vi "Floating Intake Teleop.vi"(11 "Cluster":T1) -> ()   [LabVIEW 2018]
uses:
  Support Code/Joystick Vals.ctl
  <vilib>/Rock Robotics/Network Tables/NT Read Boolean.vi
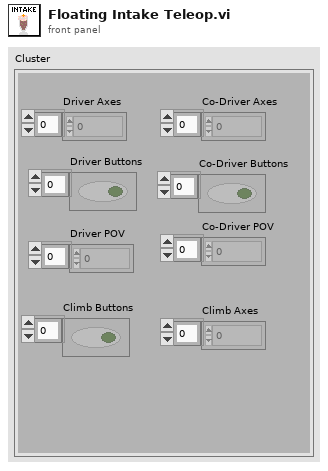
[diagram p1: front panel]
types:
  T1 = typedef "Joystick Vals.ctl" = cluster{"Driver Axes":dbl[], "Co-Driver Axes":dbl[], "Driver Buttons":bool[], "Co-Driver Buttons":bool[], "Driver POV":i16[], "Co-Driver POV":i16[], "Climb Buttons":bool[], "Climb Axes":dbl[]}
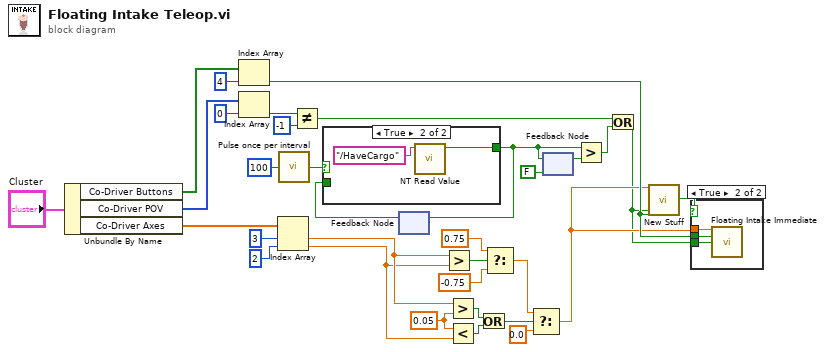
[diagram p0: block diagram]
diagram:
  w8 = 0.05 ("y")
  n1 = Unbundle By Name("Cluster") -> ("Co-Driver Buttons"=w30:bool[], "Co-Driver POV"=w26:i16[], "Co-Driver Axes"=w25:dbl[])
  n2 = Index Array(array=w30, index=4) -> (element=w15:bool)
  n3 = Index Array(array=w26, index=0) -> (element=w23:i16)
  n4 = Index Array(array=w25, index #1=3 ("index"), index #2=2 ("index")) -> (element #1=w14:dbl, element #2=w13:dbl)
  n5 = call "Pulse once per interval.vi"("Time (ms)"=u32 100 ("y")) -> ("Boolean"=w12:bool)
  n6 = Not Equal?(x=w23, y=i16 -1) -> (x != y?=w22:bool)
  n7 = feedback #1() -> (w17:bool)  [unwired: 1 in]
  n8 = case shown="True" w12 {
    tunnel: [w34 w36] -> w18
    tunnel: w17 -> [w34 _]
    frame False {
    }
    frame True {
      n9 = call-poly <vilib>:"NT Read Value.vi"("Name"="/HaveCargo") -> ("Boolean"=w36:bool)  [unwired: 9 in, 1 out]
    }
  }
  n10 = feedback-in #1(w18) -> ()
  n11 = Greater?(x=w14, y=w13) -> (0:w5:bool)
  n12 = Greater?(x=w14, y=w8) -> (0:w9:bool)
  n13 = Less?(x=w8, y=w13) -> (x < y?=w10:bool)
  n14 = Or(x=w9, y=w10) -> (x .or. y?=w11:bool)
  n15 = Select(t=0.75, s=w5, f=-0.75) -> (s? t:f=w7:dbl)
  n16 = Select(t=w7, s=w11, f=0.0) -> (s? t:f=w4:dbl)
  n17 = feedback-in #2(w18) -> ()
  n18 = feedback #2(FALSE ("Boolean")) -> (w20:bool)
  n19 = Greater?(x=w18, y=w20) -> (0:w19:bool)
  n20 = Or(x=w22, y=w19) -> (x .or. y?=w1:bool)
  n21 = call "New Stuff.vi"("Variant"=w4, "Variant 8"=w1, "Variant 7"=w15) -> ("x != y?"=w28:bool)  [unwired: 24 in]
  n22 = case shown="True" w28 {
    tunnel: w4 -> [_ w39]
    tunnel: w15 -> [_ w38]
    tunnel: w1 -> [_ w37]
    frame False {
    }
    frame True {
      n23 = call "Floating Intake Immediate.vi"("Setpoint"=w39, "Switch"=w38, "Retract"=w37) -> ()  [unwired: 12 in, 1 out]
    }
  }
